vi "Disconnect Standalone Wlan Card.vi"(8 "error in (no error)":errorcluster, 10 "USER_DUT_IP":string, 11 "_hResourceContext":u32) -> (0 "error out":errorcluster, 1 "function return":bool, 2 "USER_DUT_IP out":string, 3 "_hResourceContext out":u32)   [LabVIEW 2013, in "QCAWLAN_DLL.lvlib"]
doc: "QCA_DLL_Export bool DisconnectStandaloneWlanCard(HANDLE _hResourceContext, char* USER_DUT_IP);"
uses:
  QCAWLAN_DLL.lvlib
  QCAWLAN_DLL.dll
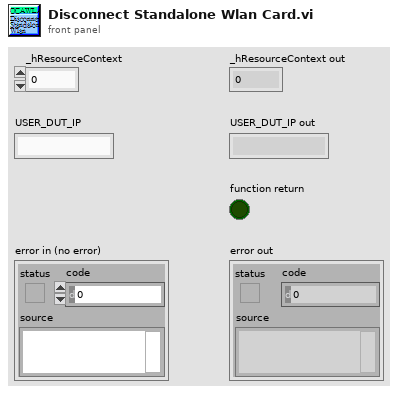
[diagram p1: front panel]
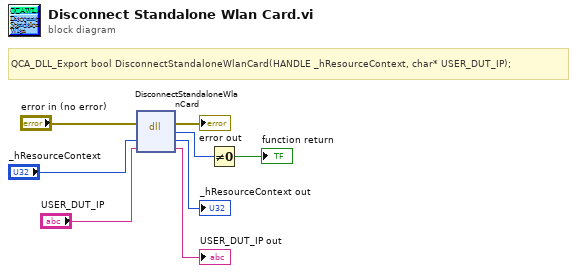
[diagram p0: block diagram]
diagram:
  # "QCA_DLL_Export bool DisconnectStandaloneWlanCard(HANDLE _hResourceContext, char* USER_DUT_IP);"
  n1 = dll-call lib="C:/Connectivity Client - MIMO/PlugIn/QCAWLAN_DLL.*" fn="DisconnectStandaloneWlanCard"(error in="error in (no error)", "_hResourceContext"="_hResourceContext", "USER_DUT_IP"="USER_DUT_IP") -> (error out=→"error out":errorcluster, w7:u8, "_hResourceContext"=→"_hResourceContext out":u32, "USER_DUT_IP"=→"USER_DUT_IP out":string)  [unwired: 2 in, 1 out]
  n2 = Not Equal To 0?(x=w7) -> (x != 0?=→"function return":bool)
